vi "Actor Core.vi"(8 "error in":errorcluster, 11 "Nested in":refnum<class "Model.lvclass">) -> (0 "error out":errorcluster, 3 "Actor out":refnum<class "Actor.lvclass">)   [LabVIEW 2015, in "Model.lvlib" / "Model.lvclass"]
doc: "(<B>Filename</B>: Actor Framework.lvlib:Actor.lvclass:Actor Core.vi)\n\nReceives messages to the actor, reacts to them, and initiates any error handling that may shut the actor down.\n\nDescendant classes may override this VI to append parallel tasks for the actor to complete while it handles messages. Overrides use the Call Parent Method node."
uses:
  Model.lvclass
  <vilib>/ActorFramework/Actor/Actor.lvclass
  <vilib>/ActorFramework/Stop Msg/Stop Msg.lvclass
  ViewController/ViewController.lvclass
  Interface/Interface.lvclass
  Model Messages/VI Operation Msg/VI Operation Msg.lvclass
  Model Messages/Update VI Information Msg/Update VI Information Msg.lvclass
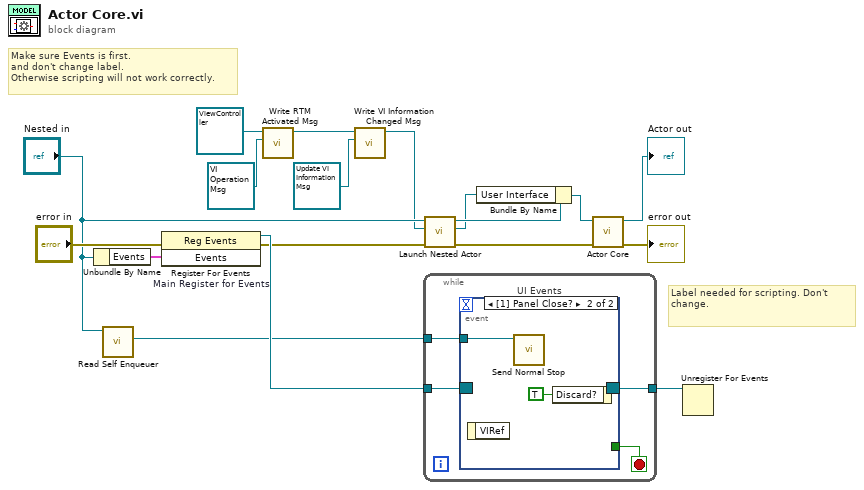
[diagram p0: block diagram]
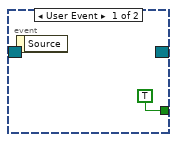
[diagram p2: hidden frame]
diagram:
  # "Label needed for scripting. Don't change."
  # "Make sure Events is first.\nand don't change label.\nOtherwise scripting will not work correctly."
  n1 = Unbundle By Name("Nested in") -> ("Events"=w15:cluster{"Stop":refnum<user-event>})
  n2 = call <vilib>:"Read Self Enqueuer.vi"("Actor"="Nested in") -> ("Self Enqueuer"=w13:refnum<class "Message Enqueuer.lvclass">)  [unwired: 10 in]
  n3 = register-events "Main Register for Events"(error in="error in", w15) -> (reference out=w16:refnum<event-registration>, error out=w11:errorcluster)  [unwired: 1 in]
  n4 = call "Write RTM Activated Msg.vi"("Interface.lvlib:RTM Activated Msg.lvclass"=refnum<class "VI Operation Msg.lvclass"> refnum ("Model.lvlib:VI Operation Msg.lvclass"), "Interface in"=refnum<class "ViewController.lvclass"> refnum ("ViewController.lvlib:ViewController.lvclass")) -> ("Interface out"=w3:refnum<class "ViewController.lvclass">)  [unwired: 9 in]
  n5 = call "Write VI Information Changed Msg.vi"("Interface.lvlib:VI Information Changed Msg.lvclass"=refnum<class "Update VI Information Msg.lvclass"> refnum ("Model.lvlib:Update VI Information Msg.lvclass"), "Interface in"=w3) -> ("Interface out"=w2:refnum<class "ViewController.lvclass">)  [unwired: 9 in]
  n6 = while {
    tunnel: w16 -> [w22]
    tunnel: [w20] -> w14
    tunnel: w13 -> [w19]
    stop <- w21 stop-if-true
    n7 = event "UI Events" shown="[1] Panel Close?" {
      selector: w22 -> [_ _]
      dyn-events: [_ _] -> w20
      timeout: _ -> [_ _]
      tunnel: [TRUE _] -> w21
      tunnel: w19 -> [_ w24]
      event User Event {
        n8 = event-data() -> ()  [unwired: 1 in, 1 out]
      }
      event Panel Close? {
        n9 = event-data() -> ()  [unwired: 1 in, 1 out]
        n10 = call <vilib>:"Send Normal Stop.vi"("Message Enqueuer"=w24) -> ()  [unwired: 10 in, 1 out]
        n11 = event-data("Discard?"=TRUE) -> ()  [unwired: 1 in, 1 out]
      }
    }
  }
  n12 = call <vilib>:"Launch Nested Actor.vi"("error in (no error)"=w11, "Nested Actor"=w2, "Caller Actor in"="Nested in") -> ("error out"=w10:errorcluster, "Nested Actor's Enqueuer"=w6:refnum<class "Message Enqueuer.lvclass">, "Caller Actor out"=w8:refnum<class "Model.lvclass">)  [unwired: 6 in]
  n13 = Bundle By Name(cluster=w8, "User Interface"=w6) -> (w7:refnum<class "Model.lvclass">)
  n14 = call-parent "Actor Core.vi"("error in"=w10, "Actor in"=w7) -> ("error out"=→"error out":errorcluster, "Actor out"=→"Actor out":refnum<class "Actor.lvclass">)  [unwired: 8 in]
  n15 = Unregister For Events(event registration refnum=w14) -> ()  [unwired: 1 in, 1 out]
